vi "Start Rx Stream.vi"(8 "error in (no error)":errorcluster, 10 "2 Ports?":bool[](array[boolean]), 11 "Refnum in":refnum<k20>[](array[refnum])) -> (0 "error out":errorcluster, 3 "Refnum out":refnum<k20>[](array[refnum]))   [LabVIEW 2016]
uses:
  <instrlib>/_niInstr/Streaming/v1/Host/Public/Start Continuous Stream.vi
  <instrlib>/_niInstr/Streaming/v1/Host/niInstr Streaming v1 Host.lvlib
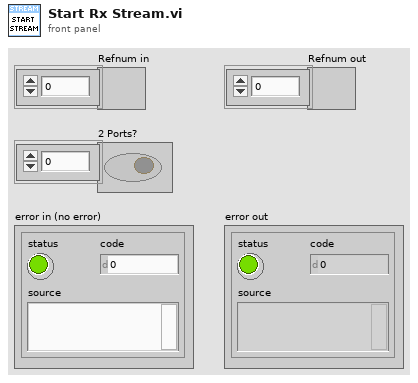
[diagram p1: front panel]
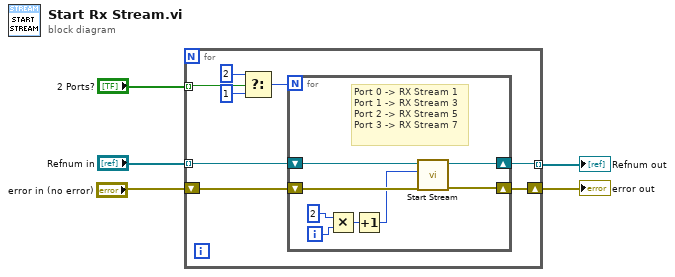
[diagram p0: block diagram]
diagram:
  n1 = for {
    tunnel: "Refnum in" -> [w12] mode=indexing
    tunnel: [w10] -> w3 mode=indexing
    shift-right: [w11] -> w4
    shift-left: "error in (no error)" -> [w13]
    tunnel: "2 Ports?" -> [w8] mode=indexing
    n2 = Select(t=2, s=w8, f=1) -> (s? t:f=w6:i32)
    n3 = for {
      N: w6 -> [_]
      shift-right: [w19] -> w10
      shift-left: w12 -> [w20]
      shift-right: [w18] -> w11
      shift-left: w13 -> [w21]
      i -> [w17]
      # "Port 0 -> RX Stream 1\nPort 1 -> RX Stream 3\nPort 2 -> RX Stream 5\nPort 3 -> RX Stream 7"
      n4 = Multiply(x=2, y=w17) -> (x*y=w15:i32)
      n5 = Increment(x=w15) -> (x+1=w14:i32)
      n6 = call-poly <instrlib>:"Start Stream.vi"("error in (no error)"=w21, "stream index"=w14, "refnum in"=w20) -> ("error out"=w18:errorcluster, "refnum out"=w19:refnum<k20>)  [unwired: 7 in]
    }
  }
  "error out" <- w4
  "Refnum out" <- w3
